vi "CRYGet Sound Device Error Informaion.vi"(11 "Error Code":i32) -> (2 "error out":errorcluster)   [LabVIEW 2013]
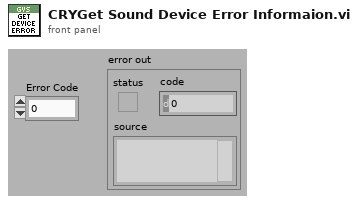
[diagram p1: front panel]
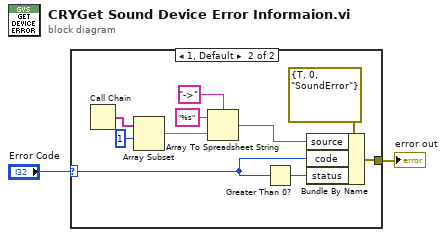
[diagram p0: block diagram]
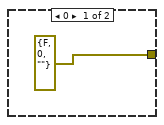
[diagram p2: hidden frame]
diagram:
  n1 = case shown="1, Default" "Error Code" {
    selector: "Error Code" -> [_ w11]
    tunnel: [errorcluster {"status"=FALSE, "code"=0, "source"=""} ("error out") w12] -> w2
    frame 0 {
    }
    frame 1, Default {
      n2 = Call Chain() -> (call chain=w7:string[])
      n3 = Array Subset(array=w7, index=1 ("Array Index")) -> (w6:string[])  [unwired: 1 in]
      n4 = Array To Spreadsheet String(delimiter (Tab)="->", array=w6, 3:"%s" ("format string")) -> (spreadsheet string=w4:string)
      n5 = Greater Than 0?(x=w11) -> (x > 0?=w10:bool)
      n6 = Bundle By Name(cluster=errorcluster {"status"=TRUE, "code"=0, "source"="SoundError"} ("error out"), "source"=w4, "code"=w11, "status"=w10) -> (w12:errorcluster)
    }
  }
  "error out" <- w2
